vi "串口.vi"() -> ()   [LabVIEW 2014]
uses:
  C:/Users/ok/Desktop/LV_HslCommunication/HslCommunication.dll
  HslCommunication.dll
panel:
  out "Content":u8[](array[numeric])
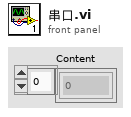
[diagram p1: front panel]
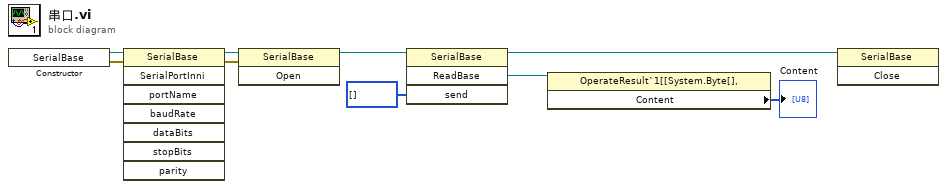
[diagram p0: block diagram]
diagram:
  n1 = constructor class="SerialBase"() -> (reference out=w8:refnum<k24>, error out=w9:errorcluster)  [unwired: 3 in, 1 out]
  n2 = invoke class="SerialBase" method="SerialPortInni"(reference=w8, error in=w9) -> (reference out=w1:refnum<k24>, error out=w7:errorcluster)  [unwired: 6 in, 6 out]
  n3 = invoke class="SerialBase" method="Open"(reference=w1, error in=w7) -> (reference out=w2:refnum<k24>)  [unwired: 1 in, 2 out]
  n4 = invoke class="SerialBase" method="ReadBase"(reference=w2, "send"=u8[] []) -> (reference out=w3:refnum<k24>, "ReadBase"=w5:refnum<k24>)  [unwired: 2 in, 2 out]
  n5 = property class="OperateResult`1[[System.Byte[],"(reference=w5) -> ("Content"=→"Content":u8[])  [unwired: 1 in, 2 out]
  n6 = invoke class="SerialBase" method="Close"(reference=w3) -> ()  [unwired: 2 in, 3 out]
